vi "Get_timebase.vi"(0 "Handle":i16, 1 "*time_interval":i16, 2 "Oversample":i16, 5 "TimeBase":i16, 7 "no_of_samples":i16, 9 "*Max_samples":i16, 11 "error in (no error)":errorcluster, 12 "*time_units":i16) -> (4 "return type":i16, 15 "error out":errorcluster)   [LabVIEW 2023]
uses:
  ps2000.dll
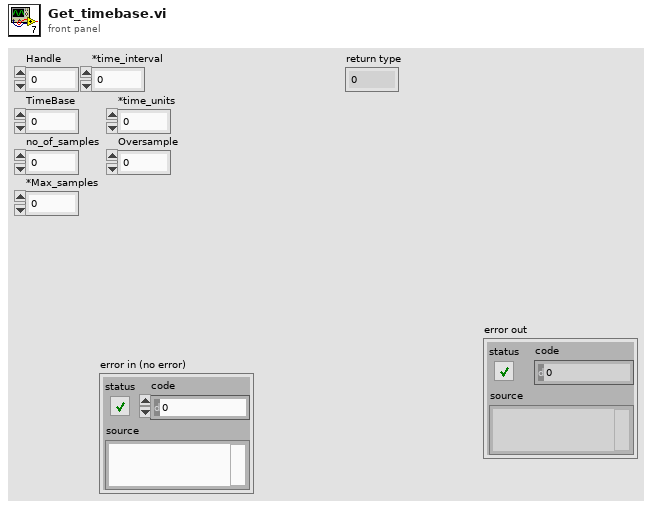
[diagram p1: front panel]
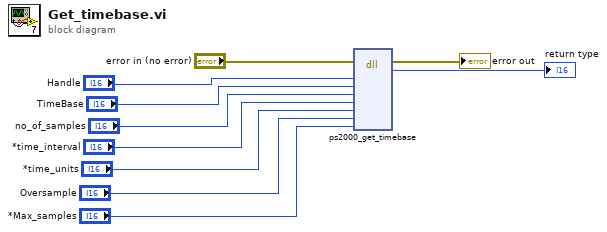
[diagram p0: block diagram]
diagram:
  n1 = dll-call lib="C:/Users/cesar/Desktop/Ps2000 libreria/PS2000.dll" fn="ps2000_get_timebase"(error in="error in (no error)", "handle"="Handle", "timebase"="TimeBase", "no_of_samples"="no_of_samples", "*time_interval"="*time_interval", "*time_units"="*time_units", "oversample"="Oversample", "*max_samples"="*Max_samples") -> (error out=→"error out":errorcluster, "return type"=→"return type":i16)  [unwired: 9 in, 1 out]
